vi "oa_Calculate CIC Decimation Filter Coefficients.vi"(6 "CIC stages":i32[](array[numeric])=[4, 6, 8], 8 "alias protect in final transition":bool, 9 "stop band attenuation":u16(ring) items=["72 dB", "96 dB", "120 dB"], 11 "decimation/interpolation factor":i32=16) -> (0 "delay":i32, 1 "lp filter settings":T1={"coefficients"=[], "factor"=1} {"coefficients" format="%.2f"}, 2 "compensation filter settings":T1={"coefficients"=[], "factor"=1} {"coefficients" format="%.2f"}, 3 "CIC Settings":cluster{"Numeric":i32, i32, i32}, 4 "interpolation factor":i32)   [LabVIEW 2017, in "SoundVib_Resampling.lvlib"]
uses:
  <vilib>/addons/Sound and Vibration/Order Analysis/Resample Order Tracking/SoundVib_Resampling.lvlib
  <vilib>/addons/_NISVFA/_Shared subVIs/Controls/OAT Decimation Filter.ctl
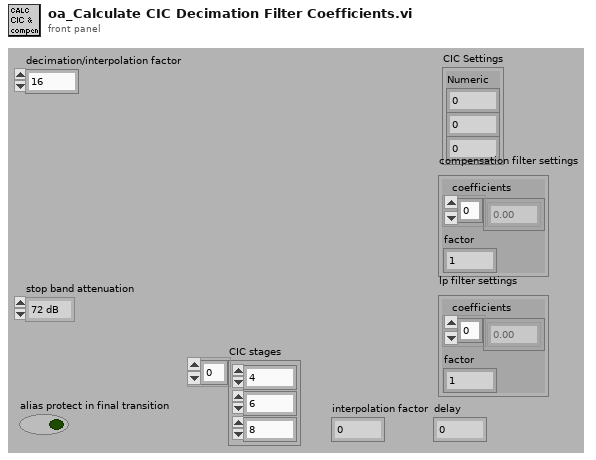
[diagram p1: front panel]
types:
  T1 = typedef "OAT Decimation Filter.ctl" = cluster{"coefficients":dbl[], "factor":i32}
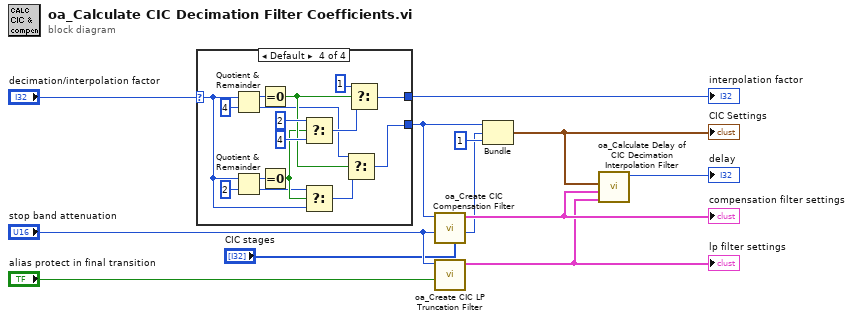
[diagram p0: block diagram]
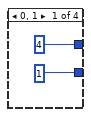
[diagram p2: hidden frame]
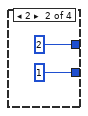
[diagram p3: hidden frame]
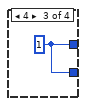
[diagram p4: hidden frame]
diagram:
  n1 = case shown="Default" "decimation/interpolation factor" {
    selector: "decimation/interpolation factor" -> [_ _ _ w18]
    tunnel: [4 2 w17 w29] -> w8
    tunnel: [1 1 w17 w19] -> w2
    frame 0, 1 {
    }
    frame 2 {
    }
    frame 4 {
      w17 = 1
    }
    frame Default {
      n2 = Quotient & Remainder(x=w18, y=4) -> (x-y*floor(x/y)=w32:i32, floor(x/y)=w21:i32)
      n3 = Quotient & Remainder(x=w18, y=2) -> (x-y*floor(x/y)=w31:i32, floor(x/y)=w20:i32)
      n4 = Equal To 0?(x=w32) -> (x = 0?=w24:bool)
      n5 = Equal To 0?(x=w31) -> (x = 0?=w22:bool)
      n6 = Select(t=2, s=w22, f=4) -> (s? t:f=w25:i32)
      n7 = Select(t=w20, s=w22, f=w18) -> (s? t:f=w23:i32)
      n8 = Select(t=w21, s=w24, f=w23) -> (s? t:f=w19:i32)
      n9 = Select(t=1, s=w24, f=w25) -> (s? t:f=w29:i32)
    }
  }
  "interpolation factor" <- w8
  n10 = call <vilib>:"oa_Create CIC Compensation Filter.vi"("CIC stages"="CIC stages", "stop band attenuation"="stop band attenuation", "decimation factor"=w2) -> ("stage"=w3:i32, "compensation filter settings"=w10:T1)  [unwired: 7 in]
  "compensation filter settings" <- w10
  n11 = call <vilib>:"oa_Create CIC LP Truncation Filter.vi"("alias protect in final transition"="alias protect in final transition", "stop band attenuation"="stop band attenuation") -> ("lp filter settings"=w9:T1)  [unwired: 9 in]
  "lp filter settings" <- w9
  n12 = Bundle("Numeric"=w2, "stage"=w3, 1) -> (w11:cluster{"Numeric":i32, "stage":i32, i32})  [unwired: 1 in]
  "CIC Settings" <- w11
  n13 = call <vilib>:"oa_Calculate Delay of CIC Decimation Interpolation Filter.vi"("lp filter settings"=w9, "compensation filter settings"=w10, "CIC decimation setting"=w11) -> ("delay"=→"delay":i32)  [unwired: 8 in]
